vi "XYMetersToVoltage.vi"(8 "error in (no error)":errorcluster, 9 "Y Coordinate":dbl, 10 "X Coordinate":dbl, 11 "Asylum_Driver in":refnum<class "Asylum_Driver.lvclass">) -> (0 "error out":errorcluster, 1 "Y Voltage":dbl, 2 "X Voltage":dbl, 3 "Asylum_Driver out":refnum<class "Asylum_Driver.lvclass">)   [LabVIEW 2019, in "Asylum_Driver.lvclass"]
uses:
  Asylum_Driver.lvclass
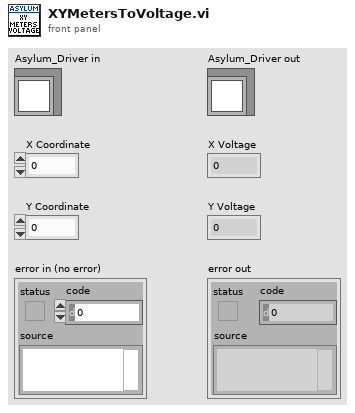
[diagram p1: front panel]
types:
  T1 = cluster{"XLVDT Sens":dbl, "YLVDT Sens":dbl, "XLVDT Offset":dbl, "YLVDT Offset":dbl}
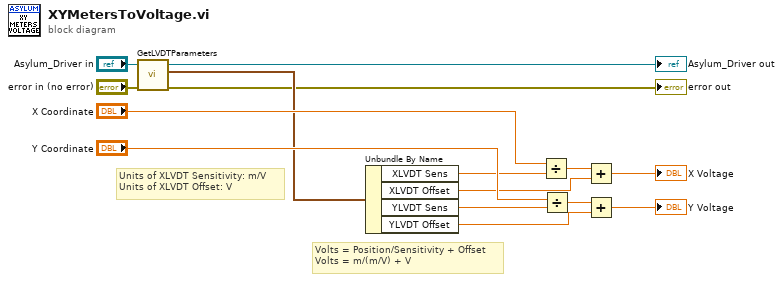
[diagram p0: block diagram]
diagram:
  # "Units of XLVDT Sensitivity: m/V\nUnits of XLVDT Offset: V"
  # "Volts = Position/Sensitivity + Offset\nVolts = m/(m/V) + V"
  n1 = call "GetLVDTParameters.vi"("error in (no error)"="error in (no error)", "Asylum_Driver in"="Asylum_Driver in") -> ("error out"=→"error out":errorcluster, "LVDT Parameters"=w3:T1, "Asylum_Driver out"=→"Asylum_Driver out":refnum<class "Asylum_Driver.lvclass">)  [unwired: 7 in]
  n2 = Unbundle By Name(w3) -> ("XLVDT Sens"=w4:dbl, "XLVDT Offset"=w6:dbl, "YLVDT Sens"=w5:dbl, "YLVDT Offset"=w9:dbl)
  n3 = Divide(x="X Coordinate", y=w4) -> (x/y=w7:dbl)
  n4 = Divide(x="Y Coordinate", y=w5) -> (x/y=w8:dbl)
  n5 = Add(x=w7, y=w6) -> (x+y=→"X Voltage":dbl)
  n6 = Add(x=w8, y=w9) -> (x+y=→"Y Voltage":dbl)
